vi "SnoInchesForSeconds.vi"(0 "Inches Desired":dbl format="%0.2f") -> (1 "Seconds for Traversal":dbl format="%0.2f", 2 "Interpolation Error":dbl format="%0.2f", 3 "In Range?":bool)   [LabVIEW 2014]
uses:
  <vilib>/Analysis/NI_AALPro.lvlib
panel:
  out "XY Graph":cluster{"Y":dbl[], "Y":dbl[]}[](graph)
  in  "Inches":dbl[](array[numeric])=[40.0, 43.0, 50.0, 51.0, 52.0, 53.0, 54.0, 55.0, 56.0, 58.0, 59.0, 60.0, 62.0, 64.0, 65.0, 68.0, 70.0, 75.0, 77.0, 80.0, 83.0, 85.0, 86.0, 90.0, 95.0, 100.0] format="%0.2f"
  in  "Seconds":dbl[](array[numeric])=[4.4, 4.5, 4.6, 4.78, 4.8, 4.8, 4.8, 4.8, 4.8, 4.85, 4.85, 4.85, 4.9, 5.0, 5.05, 5.1, 5.2, 5.25, 5.3, 5.35, 5.4, 5.45, 5.5, 5.5, 5.55, 5.6] format="%0.3f"
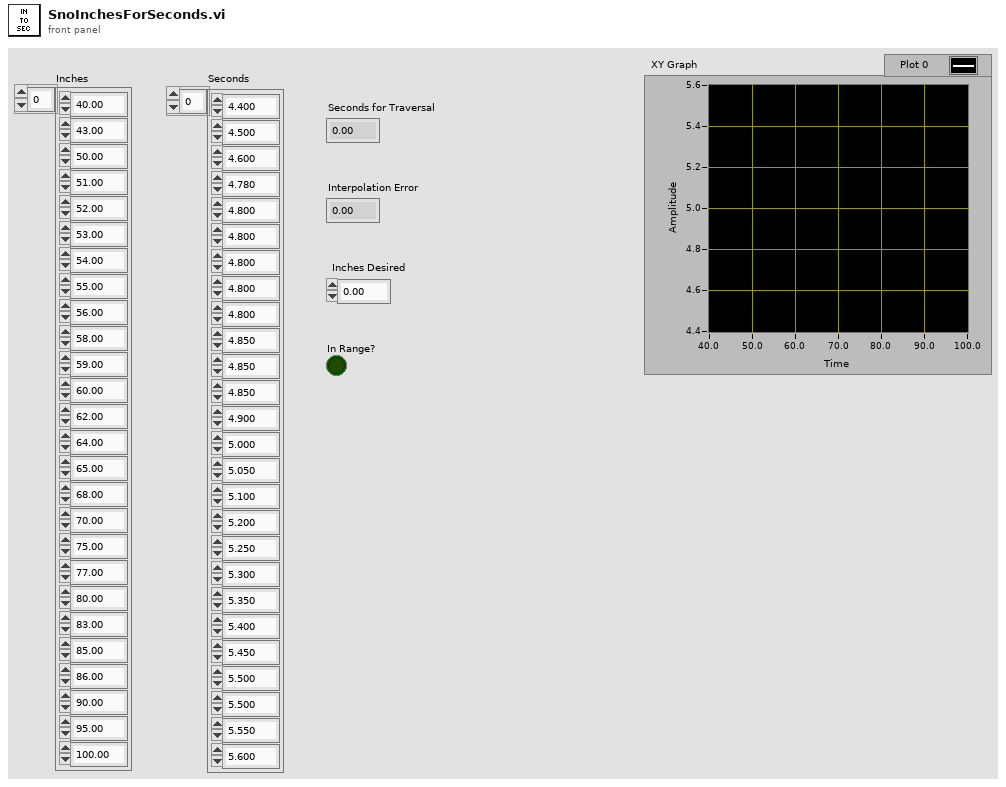
[diagram p1: front panel]
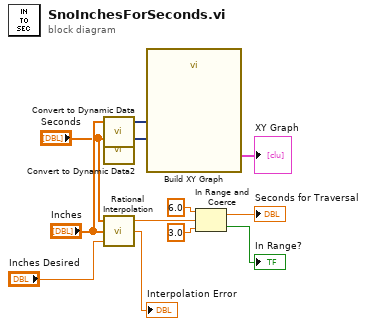
[diagram p0: block diagram]
diagram:
  n1 = call "Convert to Dynamic Data"("Array"="Inches") -> ("Dynamic Data Type"=w3:dynamicdata)  [unwired: 3 in]
  n2 = call "Convert to Dynamic Data2"("Array"="Seconds") -> ("Dynamic Data Type"=w1:dynamicdata)  [unwired: 3 in]
  n3 = call <vilib>:"Rational Interpolation.vi"("x value"="Inches Desired", "X"="Inches", "Y"="Seconds") -> ("interpolation error"=→"Interpolation Error":dbl, "interpolation value"=w7:dbl)  [unwired: 1 out]
  n4 = call "Build XY Graph"("Y Input"=w1, "X Input"=w3) -> ("XY Graph"=→"XY Graph":cluster{"X":dbl[], "Y":dbl[]}[])  [unwired: 8 in, 1 out]
  n5 = In Range and Coerce(upper limit=6.0, x=w7, lower limit=3.0) -> (coerced(x)=→"Seconds for Traversal":dbl, In Range?=→"In Range?":bool)
